vi "retrieveData.vi"(8 "error in (no error)":errorcluster, 11 "ForceSensor in":refnum<class "ForceSensor.lvclass">) -> (0 "error out":errorcluster, 3 "ForceSensor out":refnum<class "ForceSensor.lvclass">)   [LabVIEW 2013, in "ForceSensor.lvclass"]
uses:
  ForceSensor.lvclass
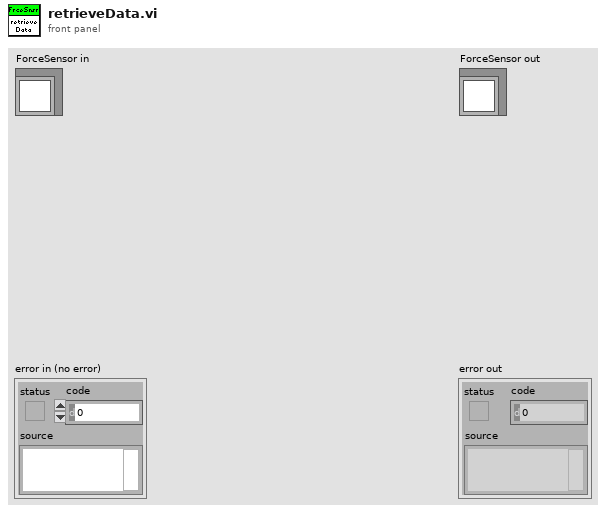
[diagram p1: front panel]
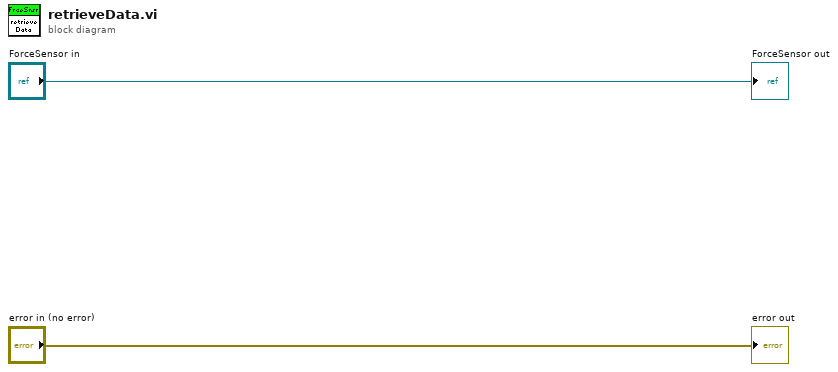
[diagram p0: block diagram]
diagram:
  "error out" <- "error in (no error)"
  "ForceSensor out" <- "ForceSensor in"
